vi "set delta level(SubVI).vi"(8 "错误输入（无错误）":errorcluster, 10 "电流（A）":dbl, 11 "VISA引用句柄输入":refnum<visa-resource-name>) -> (0 "错误输出":errorcluster, 3 "VISA引用句柄输出":refnum<visa-resource-name>)   [LabVIEW 2019, in "SubVI.lvlib"]
uses:
  SubVI.lvlib
  lib/Keithley 622x/Configure/Delta PDelta DCon Modes/Low Level/Typedefs/KE622x -- Delta PDelta Mode High Level.ctl
  lib/Keithley 622x/Keithley 622x.lvlib
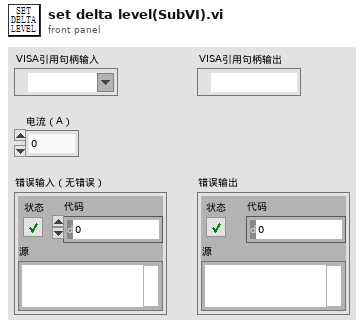
[diagram p1: front panel]
types:
  T1 = typedef "Keithley 622x.lvlib/KE622x -- Delta PDelta Mode High Level.ctl" = dbl
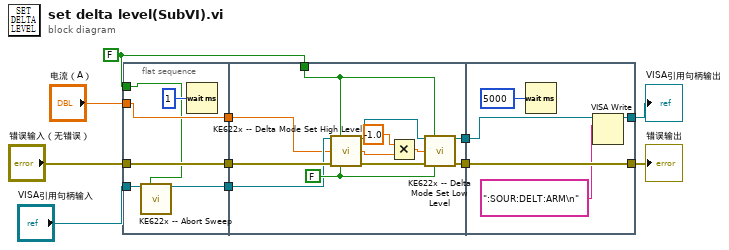
[diagram p0: block diagram]
diagram:
  w1 = FALSE ("Check For SCPI Errors? (T)")
  n1 = flat-sequence {
    tunnel: "电流（A）" -> [w16]
    tunnel: "VISA引用句柄输入" -> [w14]
    tunnel: "错误输入（无错误）" -> [w17]
    tunnel: [w17] -> w6
    tunnel: [w16] -> w5
    tunnel: [w13] -> w2
    tunnel: w1 -> [w12]
    tunnel: w6 -> [w29]
    tunnel: w5 -> [w18]
    tunnel: [w27] -> w4
    tunnel: [w25] -> w3
    tunnel: w2 -> [w24]
    tunnel: w1 -> [w19]
    tunnel: [w30] -> w9
    tunnel: [w34] -> w10
    tunnel: w4 -> [w34]
    tunnel: w3 -> [w31]
    frame #0 {
      n2 = call "KE622x -- Abort Sweep.vi"("Resource In"=w14, "Check For SCPI Errors? (T)"=w12) -> ("Resource Out (dupl)"=w13:refnum<visa-resource-name>)  [unwired: 12 in, 1 out]
      n3 = Wait (ms)(milliseconds to wait=u32 1) -> ()  [unwired: 1 out]
    }
    frame #1 {
      w28 = FALSE
      n4 = call "KE622x -- Delta Mode Set High Level.vi"("Resource In"=w24, "Check For SCPI Errors? (T)"=w19, "High Level In (A)"=w18, "error in (no error)"=w29, "Read Back Set Value? (T)"=w28) -> ("Resource Out (dupl)"=w20:refnum<visa-resource-name>, "High Level Out (A)"=w21:T1, "error out"=w26:errorcluster)  [unwired: 8 in]
      n5 = Multiply(x=T1 -1.0, y=w21) -> (x*y=w23:T1)
      n6 = call "KE622x -- Delta Mode Set Low Level.vi"("Resource In"=w20, "Check For SCPI Errors? (T)"=w19, "Low Level In (A)"=w23, "error in (no error)"=w26, "Read Back Set Value? (T)"=w28) -> ("Resource Out (dupl)"=w25:refnum<visa-resource-name>, "error out"=w27:errorcluster)  [unwired: 8 in, 1 out]
    }
    frame #2 {
      n7 = Wait (ms)(milliseconds to wait=u32 5000) -> ()  [unwired: 1 out]
      n8 = VISA Write(VISA resource name=w31, write buffer=":SOUR:DELT:ARM\n" ("format string")) -> (VISA resource name out=w30:refnum<visa-resource-name>)  [unwired: 1 in, 2 out]
    }
  }
  "错误输出" <- w10
  "VISA引用句柄输出" <- w9
